vi "外设配置对话框.vi"() -> ()   [LabVIEW 2016, in "斯坦道通用流路CODmn.lvlib"]
uses:
  <vilib>/Utility/miscctls.llb/LVPointTypeDef.ctl
panel:
  out "选项卡控件":enum32{"V3 A版", "V3 A1版", "V3 B版"}(tab)
  in  "A版外设配置":T1 {"阀方向" items=["顺时针", "逆时针", "就近"]; "总氮x公式0" items=["0", "1"]; "光谱仪类型" items=["1型", "2型", "3型", "2型氙灯联控"]; "泵阀量" items=["9通"=9, "10通"=10, "12通"=12]; "泵类型" items=["1型", "2型", "sy04型+旋转阀"]}
  in  "A1版外设配置":T2 {"总氮x公式0" items=["0", "1"]; "光谱仪类型" items=["1型", "2型", "3型", "2型氙灯联控"]; "泵阀量" items=["9通"=9, "10通"=10, "12通"=12]; "泵类型" items=["1型", "2型", "sy04型+旋转阀"]}
  in  "B版外设配置":T3 {"阀型号" items=["垦拓10通阀"]; "总氮x公式0" items=["0", "1"]; "光谱仪类型" items=["1型", "2型", "3型", "2型氙灯联控"]; "泵类型" items=["润泽注射泵", "垦拓注射泵"]}
  in  "关闭":bool
  in  "保存":bool
  in  "读取":bool
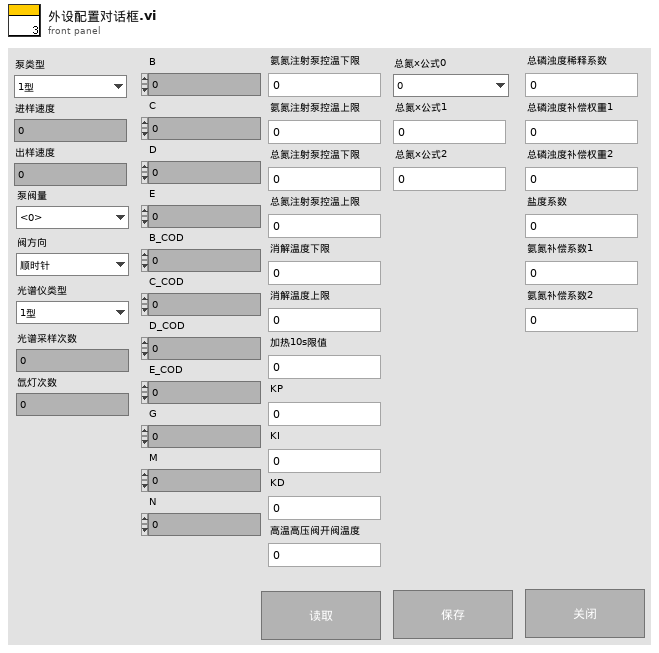
[diagram p1: front panel]
types:
  T1 = typedef "斯坦道通用流路CODmn.lvlib/V3 A版外设参数.ctl" = cluster{"泵类型":u8, "进样速度":u32, "出样速度":u32, "泵阀量":u8, "阀方向":u8, "光谱仪类型":u8, "光谱采样次数":u8, "氙灯次数":u8, "B":u16, "C":u16, "D":u16, "E":u16, "B_COD":u16, "C_COD":u16, "D_COD":u16, "E_COD":u16, "G":u16, "M":u16, "N":u16, "氨氮注射泵控温下限":sgl, "氨氮注射泵控温上限":sgl, "总氮注射泵控温下限":sgl, "总氮注射泵控温上限":sgl, "消解温度下限":sgl, "消解温度上限":sgl, "加热10s限值":sgl, "KP":sgl, "KI":sgl, "KD":sgl, "高温高压阀开阀温度":sgl, "总氮x公式0":u8, "总氮x公式1":sgl, "总氮x公式2":sgl, "总磷浊度稀释系数":sgl, "总磷浊度补偿权重1":sgl, "总磷浊度补偿权重2":sgl, "盐度系数":sgl, "氨氮补偿系数1":sgl, "氨氮补偿系数2":sgl}
  T2 = typedef "斯坦道通用流路CODmn.lvlib/V3 A1版外设参数.ctl" = cluster{"泵类型":u8, "进样速度":u32, "出样速度":u32, "泵阀量":u8, "光谱仪类型":u8, "光谱采样次数":u8, "氙灯次数":u8, "B":u16, "C":u16, "D":u16, "E":u16, "B_COD":u16, "C_COD":u16, "D_COD":u16, "E_COD":u16, "G":u16, "M":u16, "N":u16, "氨氮注射泵控温下限":sgl, "氨氮注射泵控温上限":sgl, "总氮注射泵控温下限":sgl, "总氮注射泵控温上限":sgl, "消解温度下限":sgl, "消解温度上限":sgl, "加热10s限值":sgl, "高温高压阀开阀温度":sgl, "总氮x公式0":u8, "总氮x公式1":sgl, "总氮x公式2":sgl, "总磷浊度稀释系数":sgl, "总磷浊度补偿权重1":sgl, "总磷浊度补偿权重2":sgl, "盐度系数":sgl, "氨氮补偿系数1":sgl, "氨氮补偿系数2":sgl}
  T3 = typedef "斯坦道通用流路CODmn.lvlib/V3 B版外设参数.ctl" = cluster{"泵类型":u8, "注射泵正常速度":u32, "注射泵慢速":u32, "阀型号":u8, "res":u8, "光谱仪类型":u8, "光谱采样次数":u8, "氙灯次数":u8, "B":u16, "C":u16, "D":u16, "E":u16, "B_COD":u16, "C_COD":u16, "D_COD":u16, "E_COD":u16, "G":u16, "M":u16, "N":u16, "降温下限":sgl, "降温上限":sgl, "恒温温度下限":sgl, "恒温温度上限":sgl, "消解温度下限":sgl, "消解温度上限":sgl, "加热10s限值":sgl, "KP":sgl, "KI":sgl, "KD":sgl, "高温高压阀开阀温度":sgl, "总氮x公式0":u8, "总氮x公式1":sgl, "总氮x公式2":sgl, "总磷浊度稀释系数":sgl, "总磷浊度补偿权重1":sgl, "总磷浊度补偿权重2":sgl, "盐度系数":sgl, "氨氮补偿系数1":sgl, "氨氮补偿系数2":sgl, "缺试剂传感器阈值":u16}
  T4 = typedef "LVPointTypeDef.ctl" = cluster{"Horizontal":i16, "Vertical":i16}
  T5 = typedef "SingleStepTestV3.lvlib/SingleStepTestV3.lvclass/仪器版本.ctl" = enum16{"A版", "B版", "A1版"}
  T6 = typedef "操作日志字段定义.ctl" = cluster{"时间":timestamp, "参数":string, "日志信息":string, "流程参数":string}
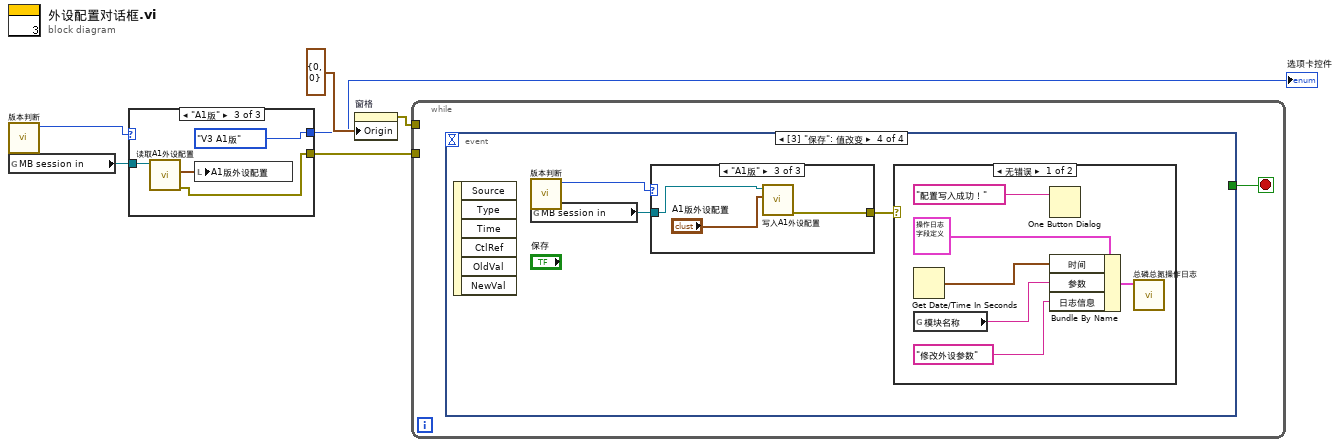
[diagram p0: block diagram]
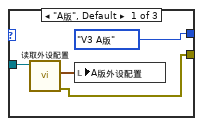
[diagram p2: hidden frame]
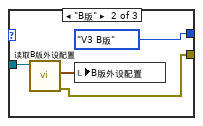
[diagram p3: hidden frame]
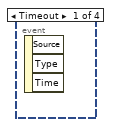
[diagram p4: hidden frame]
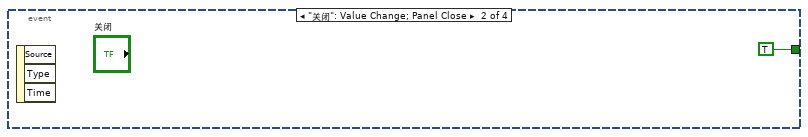
[diagram p5: hidden frame]
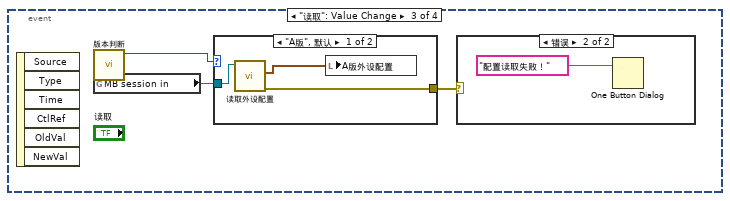
[diagram p6: hidden frame]
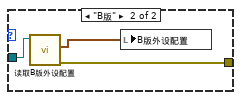
[diagram p8: hidden frame]
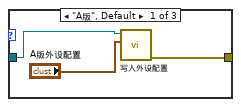
[diagram p10: hidden frame]
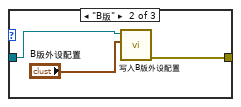
[diagram p11: hidden frame]
diagram:
  n1 = call "版本判断.vi"() -> ("仪器版本"=w3:T5)  [unwired: 11 in]
  n2 = global read "VAR总磷总氮全局变量.vi" "MB session in"() -> (w2:refnum<class "MB_Master.lvclass">)
  n3 = case shown="\"A1版\"" w3 {
    tunnel: [w10 w13 w17] -> w6
    tunnel: w2 -> [w8 w14 w18]
    tunnel: [enum32{"V3 A版", "V3 A1版", "V3 B版"}."V3 A版" ("选项卡控件") enum32{"V3 A版", "V3 A1版", "V3 B版"}."V3 B版" ("选项卡控件") enum32{"V3 A版", "V3 A1版", "V3 B版"}."V3 A1版" ("选项卡控件")] -> w1
    frame "A版", Default {
      n4 = call "读取外设配置.vi"("MB session in"=w8) -> ("error out"=w10:errorcluster, "外设配置"=w9:T1)  [unwired: 8 in, 1 out]
      n5 = local write "A版外设配置"(w9) -> ()
    }
    frame "B版" {
      n6 = call "读取B版外设配置.vi"("MB session in"=w14) -> ("error out"=w13:errorcluster, "外设配置"=w12:T3)  [unwired: 8 in, 1 out]
      n7 = local write "B版外设配置"(w12) -> ()
    }
    frame "A1版" {
      n8 = call "读取A1外设配置.vi"("MB session in"=w18) -> ("error out"=w17:errorcluster, "外设配置"=w15:T2)  [unwired: 8 in, 1 out]
      n9 = local write "A1版外设配置"(w15) -> ()
    }
  }
  "选项卡控件" <- w1
  n10 = property on="窗格" class="Pane"("Origin"=T4 {"Horizontal"=0, "Vertical"=0} ("原点")) -> (error out=w4:errorcluster)  [unwired: 2 in, 1 out]
  n11 = while {
    tunnel: w6 -> [_]
    tunnel: w4 -> [_]
    stop <- w19 stop-if-true
    n12 = event shown="[3] \"保存\": 值改变" {
      selector: _ -> [_ _ _ _]
      dyn-events: _ -> [_ _ _ _]
      timeout: _ -> [_ _ _ _]
      tunnel: [_ TRUE _ _] -> w19
      event Timeout {
        n13 = event-data() -> ()  [unwired: 1 in, 3 out]
      }
      event "关闭": Value Change; Panel Close {
        n14 = event-data() -> ()  [unwired: 1 in, 3 out]
      }
      event "读取": Value Change {
        n15 = event-data() -> ()  [unwired: 1 in, 6 out]
        n16 = call "版本判断.vi"() -> ("仪器版本"=w23:T5)  [unwired: 11 in]
        n17 = global read "VAR总磷总氮全局变量.vi" "MB session in"() -> (w22:refnum<class "MB_Master.lvclass">)
        n18 = case shown="\"A版\", 默认" w23 {
          tunnel: [w27 w29] -> w21
          tunnel: w22 -> [w25 w30]
          frame "A版", Default {
            n19 = call "读取外设配置.vi"("MB session in"=w25) -> ("error out"=w27:errorcluster, "外设配置"=w26:T1)  [unwired: 8 in, 1 out]
            n20 = local write "A版外设配置"(w26) -> ()
          }
          frame "B版" {
            n21 = call "读取B版外设配置.vi"("MB session in"=w30) -> ("error out"=w29:errorcluster, "外设配置"=w28:T3)  [unwired: 8 in, 1 out]
            n22 = local write "B版外设配置"(w28) -> ()
          }
        }
        n23 = case shown="错误" w21 {
          frame No Error {
          }
          frame Error {
            n24 = One Button Dialog(message="配置读取失败！") -> ()  [unwired: 1 in, 1 out]
          }
        }
      }
      event "保存": Value Change {
        n25 = event-data() -> ()  [unwired: 1 in, 6 out]
        n26 = call "版本判断.vi"() -> ("仪器版本"=w32:T5)  [unwired: 11 in]
        n27 = global read "VAR总磷总氮全局变量.vi" "MB session in"() -> (w33:refnum<class "MB_Master.lvclass">)
        n28 = case shown="\"A1版\"" w32 {
          tunnel: [w42 w43 w47] -> w31
          tunnel: w33 -> [w41 w44 w48]
          frame "A版", Default {
            n29 = call "写入外设配置.vi"("外设配置"="A版外设配置", "MB session in"=w41) -> ("error out"=w42:errorcluster)  [unwired: 8 in, 1 out]
          }
          frame "B版" {
            n30 = call "写入B版外设配置.vi"("外设配置"="B版外设配置", "MB session in"=w44) -> ("error out"=w43:errorcluster)  [unwired: 8 in, 1 out]
          }
          frame "A1版" {
            n31 = call "写入A1外设配置.vi"("外设配置"="A1版外设配置", "MB session in"=w48) -> ("error out"=w47:errorcluster)  [unwired: 8 in, 1 out]
          }
        }
        n32 = case shown="无错误" w31 {
          frame No Error {
            n33 = Get Date/Time In Seconds() -> (seconds since 1Jan1904=w36:timestamp)
            n34 = global read "VAR总磷总氮全局变量.vi" "模块名称"() -> (w34:string)
            n35 = One Button Dialog(message="配置写入成功！") -> ()  [unwired: 1 in, 1 out]
            n36 = Bundle By Name(cluster=T6 {"时间"=timestamp(0 s since 1904-01-01), "参数"="", "日志信息"="", "流程参数"=""} ("data in"), "时间"=w36, "参数"=w34, "日志信息"="修改外设参数") -> (w37:T6)
            n37 = call "总磷总氮操作日志.vi"("data in"=w37) -> ()  [unwired: 10 in, 1 out]
          }
          frame Error {
          }
        }
      }
    }
  }
